vi "SetLocal.vi"(8 "Error In":errorcluster, 10 "Local?":bool, 11 "Keithley 7001 In":refnum<visa-resource-name>) -> (0 "Error Out":errorcluster, 3 "Keithley 7001 Out":refnum<visa-resource-name>)   [LabVIEW 2012, in "Keithley-7001.lvlib"]
uses:
  Keithley-7001.lvlib
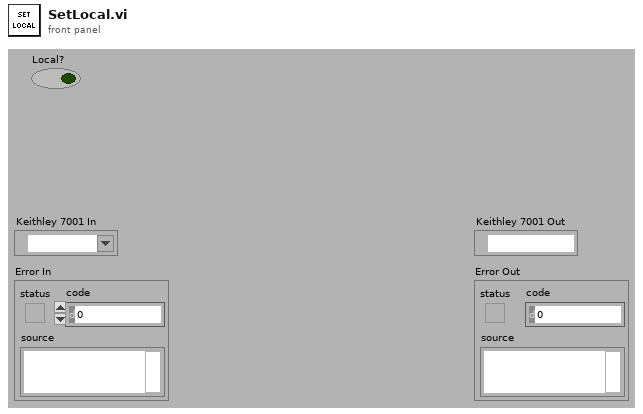
[diagram p1: front panel]
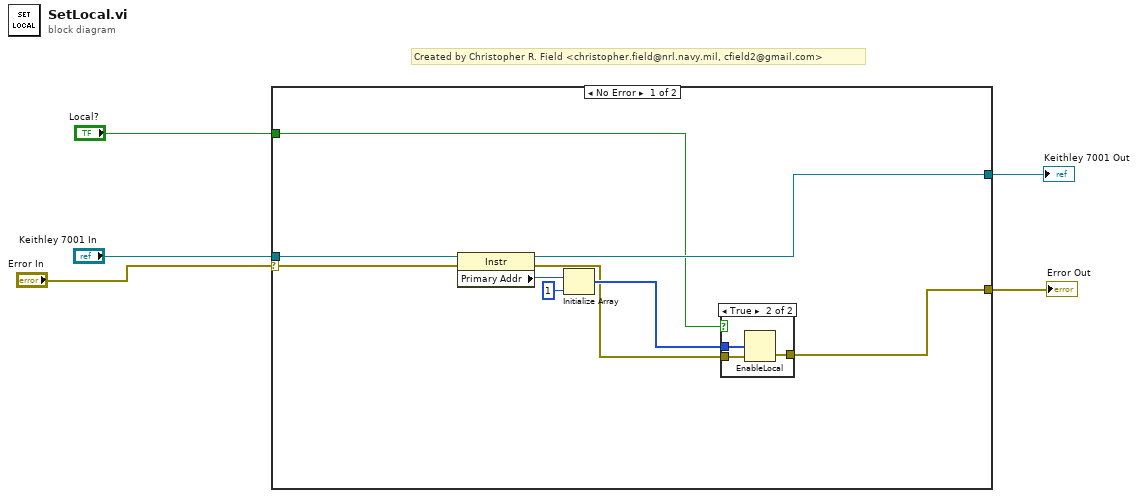
[diagram p0: block diagram]
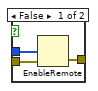
[diagram p2: hidden frame]
diagram:
  # "Created by Christopher R. Field <christopher.field@nrl.navy.mil, cfield2@gmail.com>"
  n1 = case shown="No Error" "Error In" {
    selector: "Error In" -> [w6 w21]
    tunnel: "Keithley 7001 In" -> [w14 w22]
    tunnel: [w13 w22] -> w4
    tunnel: [w8 w21] -> w3
    tunnel: "Local?" -> [w7 _]
    frame No Error {
      n2 = property class="Instr"(reference=w14, error in=w6) -> (reference out=w13:refnum<visa-resource-name>, error out=w9:errorcluster, "Primary Addr"=w12:u16)
      n3 = Initialize Array(w12, u8 1 ("dimension size")) -> (w10:u16[])
      n4 = case shown="True" w7 {
        tunnel: w10 -> [w17 w20]
        tunnel: w9 -> [w16 w19]
        tunnel: [w15 w18] -> w8
        frame False {
          n5 = EnableRemote(2:w16, 3:w17) -> (0:w15:errorcluster)  [unwired: 1 in, 1 out]
        }
        frame True {
          n6 = EnableLocal(2:w19, 3:w20) -> (0:w18:errorcluster)  [unwired: 1 in, 1 out]
        }
      }
    }
    frame Error {
    }
  }
  "Keithley 7001 Out" <- w4
  "Error Out" <- w3
